vi "Format Expand Structure.vi"(5 "Enable? (T)":bool=TRUE, 7 "Title (Click here to expand...)":string="Click here to expand...", 8 "Error in":errorcluster caption="Error in (no error)", 11 "Content":string) -> (0 "Error out":errorcluster, 3 "Expand String":string)   [LabVIEW 2023, in "Confluence Formatting.lvlib"]
uses:
  Confluence Formatting.lvlib
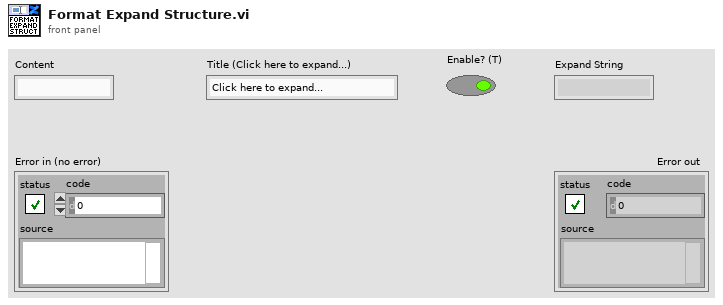
[diagram p1: front panel]
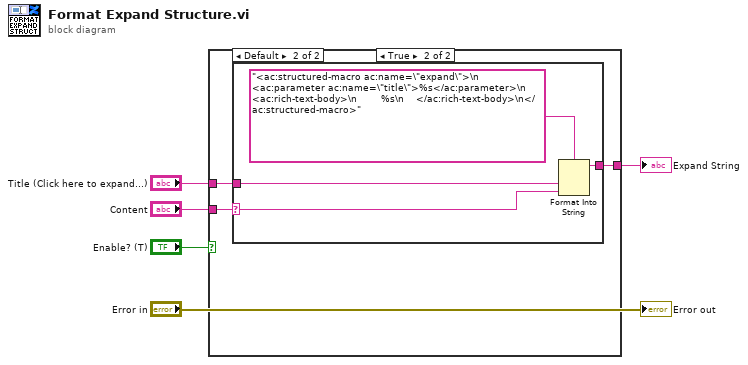
[diagram p0: block diagram]
diagram:
  n1 = case shown="True" "Enable? (T)" {
    tunnel: "Title (Click here to expand...)" -> [_ w9]
    tunnel: "Content" -> [w6 w8]
    tunnel: [w6 w7] -> w2
    frame False {
    }
    frame True {
      n2 = case shown="Default" w8 {
        selector: w8 -> [w10 w12]
        tunnel: w9 -> [_ w13]
        tunnel: [w10 w11] -> w7
        frame "" {
        }
        frame Default {
          n3 = Format Into String(format string="<ac:structured-macro ac:name=\"expand\">\n    <ac:parameter ac:name=\"title\">%s</ac:parameter>\n    <ac:rich-text-body>\n        %s\n    </ac:rich-text-body>\n</ac:structured-macro>", w13, w12) -> (resulting string=w11:string)  [unwired: 2 in, 1 out]
        }
      }
    }
  }
  "Expand String" <- w2
  "Error out" <- "Error in"
